vi "CreateErrorControls.vi"(8 "error in (no error)":errorcluster, 11 "VI in":refnum<vi>) -> (0 "error out":errorcluster, 2 "Control terminals on top-level":refnum<vi>[](array[refnum]), 3 "VI out (dup)":refnum<vi>, 4 "Error terminals":T1)   [LabVIEW 2017, in "ErrorStructureDrawer.lvlib"]
doc: "Checks if an error control and error indicator exist. If so, gets a reference to it/them. Otherwise, creates and positions (within front panel) an error control and/or error indicator."
uses:
  ErrorStructureDrawer.lvlib
  Controls/ErrorTerminals.ctl
  <vilib>/Utility/traverseref.llb/TRef TravTarget.ctl
  <vilib>/Utility/miscctls.llb/LVPointTypeDef.ctl
  <vilib>/Utility/miscctls.llb/LVPositionTypeDef.ctl
  GetErrorControlVertSpacingFP.vi
  GetErrorControlPath.vi
  GetErrorControlHorizSpacingFP.vi
  GetErrorIndicatorPath.vi
  <vilib>/Utility/traverseref.llb/VI Scripting - Traverse.lvlib
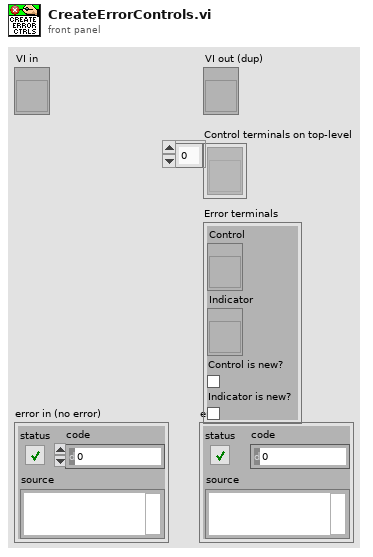
[diagram p1: front panel]
types:
  T1 = typedef "ErrorStructureDrawer.lvlib/ErrorTerminals.ctl" = cluster{"Control":refnum<vi>, "Indicator":refnum<vi>, "Control is new?":bool, "Indicator is new?":bool}
  T2 = typedef "LVPositionTypeDef.ctl" = cluster{"Left":i32, "Top":i32}
  T3 = typedef "LVPointTypeDef.ctl" = cluster{"Horizontal":i16, "Vertical":i16}
  T4 = typedef "TRef TravTarget.ctl" = enum16{"FP", "BD", "Other"}
  T5 = typedef "LVBoundsTypeDef.ctl" = cluster{"Width":u32, "Height":u32}
  T6 = typedef "LVRectTypeDef.ctl" = cluster{"Left":i16, "Top":i16, "Right":i16, "Bottom":i16}
  T7 = cluster{"Left":i32, "Top":i32, "Right":i32, "Bottom":i32}
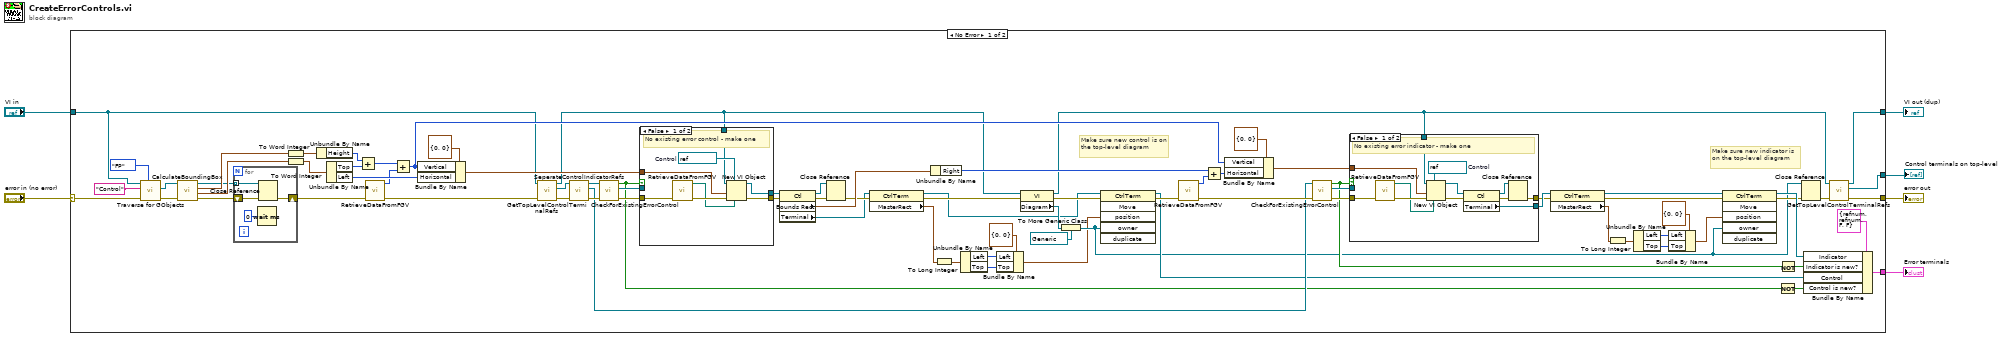
[diagram p0: block diagram]
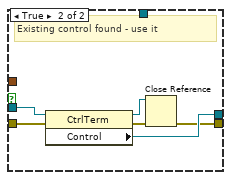
[diagram p3: hidden frame]
diagram:
  n1 = case shown="No Error" "error in (no error)" {
    selector: "error in (no error)" -> [w56 w122]
    tunnel: "VI in" -> [w50 w121]
    tunnel: [w59 w122] -> w5
    tunnel: [w63 _] -> w4
    tunnel: [w57 w121] -> w2
    tunnel: [w58 _] -> w1
    frame No Error {
      # "Make sure new indicator is on the top-level diagram"
      # "Make sure new control is on the top-level diagram"
      n2 = call <vilib>:"Traverse for GObjects.vi"("Traverse Target"=TRef_TravTarget."FP", "error in (no error)"=w56, "Class Name"="Control", "VI Refnum"=w50) -> ("error out"=w71:errorcluster, "References"=w86:refnum<vi>[])  [unwired: 4 in, 2 out]
      n3 = call "CalculateBoundingBox.vi"("error in (no error)"=w71, "Items"=w86) -> ("error out"=w67:errorcluster, "Current bounding box position"=w80:cluster{"Left":i32, "Top":i32}, "Size of bounding box for items"=w82:T5, "Items out (dup)"=w68:refnum<vi>[])  [unwired: 6 in]
      n4 = for {
        tunnel: w68 -> [w120] mode=indexing
        shift-right: [w118] -> w60
        shift-left: w67 -> [w119]
        n5 = Wait (ms)(milliseconds to wait=u32 0) -> ()  [unwired: 1 out]
        n6 = Close Reference(reference=w120, error in (no error)=w119) -> (error out=w118:errorcluster)
      }
      n7 = To Word Integer(number=w82) -> (16bit integer=w81:cluster{"Width":i16, "Height":i16})
      n8 = To Word Integer(number=w80) -> (16bit integer=w79:cluster{"Left":i16, "Top":i16})
      n9 = Unbundle By Name(w81) -> ("Height"=w83:i16)
      n10 = Unbundle By Name(w79) -> ("Top"=w78:i16, "Left"=w77:i16)
      n11 = Add(x=w83, y=w78) -> (x+y=w76:i16)
      n12 = call-poly "RetrieveDataFromFGV.vi"("error in (no error)"=w60) -> ("error out"=w51:errorcluster, "Error control vertical spacing from existing FP items"=w61:i16)  [unwired: 9 in]
      n13 = Add(x=w76, y=w61) -> (x+y=w72:i16)
      n14 = Bundle By Name(cluster=T3 {"Horizontal"=0, "Vertical"=0} ("location"), "Vertical"=w72, "Horizontal"=w77) -> (w84:T3)
      n15 = call "GetTopLevelControlTerminalRefs.vi"("error in (no error)"=w51, "VI ref in"=w50) -> ("error out"=w55:errorcluster, "Control terminals on top-level"=w54:refnum<vi>[], "VI ref out (dup)"=w35:refnum<vi>)  [unwired: 7 in]
      n16 = call "SeperateControlIndicatorRefs.vi"("error in (no error)"=w55, "Terminal references"=w54) -> ("error out"=w53:errorcluster, "Indicator references"=w43:refnum<vi>[], "Control references"=w52:refnum<vi>[])  [unwired: 7 in]
      n17 = call "CheckForExistingErrorControl.vi"("error in (no error)"=w53, "Control terminals to check"=w52) -> ("error out"=w49:errorcluster, "Error control ref"=w48:refnum<vi>, "Error control found?"=w42:bool)  [unwired: 7 in]
      n18 = case shown="False" w42 {
        tunnel: w84 -> [w109 _]
        tunnel: [w108 w114] -> w75
        tunnel: [w107 w112] -> w70
        tunnel: w49 -> [w104 w116]
        tunnel: w35 -> [w103 _]
        tunnel: w48 -> [_ w115]
        frame False {
          w110 = refnum<vi> refnum  # Control
          # "No existing error control - make one"
          n19 = call-poly "RetrieveDataFromFGV.vi"("error in (no error)"=w104) -> ("error out"=w106:errorcluster, "Error control path"=w105:path)  [unwired: 9 in]
          n20 = New VI Object(vi object class=w110, owner refnum=w103, position/next to=w109, 6:w105, 8:w106) -> (object refnum=w108:refnum<vi>, 0:w107:errorcluster)  [unwired: 3 in]
        }
        frame True {
          # "Existing control found - use it"
          n21 = property class="CtrlTerm"(reference=w115, error in=w116) -> (reference out=w111:refnum<vi>, error out=w113:errorcluster, "Control"=w114:refnum<vi>)
          n22 = Close Reference(reference=w111, error in (no error)=w113) -> (error out=w112:errorcluster)
        }
      }
      n23 = property class="Ctl"(reference=w75, error in=w70) -> (reference out=w65:refnum<vi>, error out=w66:errorcluster, "Bounds Rect"=w22:T6, "Terminal"=w10:refnum<vi>)
      n24 = Close Reference(reference=w65, error in (no error)=w66) -> (error out=w11:errorcluster)
      n25 = property class="CtrlTerm"(reference=w10, error in=w11) -> (reference out=w7:refnum<vi>, error out=w8:errorcluster, "MasterRect"=w9:T6)
      n26 = Unbundle By Name(w22) -> ("Right"=w47:i16)
      n27 = To Long Integer(number=w9) -> (32bit integer=w23:T7)
      n28 = Unbundle By Name(w23) -> ("Left"=w25:i32, "Top"=w24:i32)
      n29 = Bundle By Name(cluster=T2 {"Left"=0, "Top"=0} ("position"), "Left"=w25, "Top"=w24) -> (w26:T2)
      n30 = property class="VI"(reference=w35, error in=w8) -> (reference out=w34:refnum<vi>, error out=w36:errorcluster, "Diagram"=w33:refnum<vi>)
      n31 = To More Generic Class(target class=refnum<vi> refnum ("owner"), reference=w33) -> (generic class reference=w28:refnum<vi>)
      n32 = invoke class="CtrlTerm" method="Move"(reference=w7, error in=w36, "position"=w26, "owner"=w28) -> (reference out=w37:refnum<vi>, error out=w38:errorcluster)  [unwired: 2 in, 4 out]
      n33 = call-poly "RetrieveDataFromFGV.vi"("error in (no error)"=w38) -> ("error out"=w46:errorcluster, "Error control-indicator horizontal spacing on FP"=w62:i16)  [unwired: 9 in]
      n34 = Add(x=w47, y=w62) -> (x+y=w69:i16)
      n35 = Bundle By Name(cluster=T3 {"Horizontal"=0, "Vertical"=0} ("location"), "Vertical"=w72, "Horizontal"=w69) -> (w73:T3)
      n36 = call "CheckForExistingErrorControl.vi"("error in (no error)"=w46, "Control terminals to check"=w43) -> ("error out"=w45:errorcluster, "Error control ref"=w44:refnum<vi>, "Error control found?"=w40:bool)  [unwired: 7 in]
      n37 = case shown="False" w40 {
        tunnel: w73 -> [w98 _]
        tunnel: [w94 w101] -> w21
        tunnel: w45 -> [w91 w102]
        tunnel: [w90 w102] -> w20
        tunnel: w34 -> [w89 _]
        tunnel: w44 -> [_ w101]
        frame False {
          w100 = refnum<vi> refnum  # Control
          # "No existing error indicator - make one"
          n38 = call-poly "RetrieveDataFromFGV.vi"("error in (no error)"=w91) -> ("error out"=w93:errorcluster, "Error indicator path"=w92:path)  [unwired: 9 in]
          n39 = New VI Object(vi object class=w100, owner refnum=w89, position/next to=w98, 6:w92, 8:w93) -> (object refnum=w96:refnum<vi>, 0:w99:errorcluster)  [unwired: 3 in]
          n40 = property class="Ctl"(reference=w96, error in=w99) -> (reference out=w95:refnum<vi>, error out=w97:errorcluster, "Terminal"=w94:refnum<vi>)
          n41 = Close Reference(reference=w95, error in (no error)=w97) -> (error out=w90:errorcluster)
        }
        frame True {
          # "Existing indicator found - use it"
        }
      }
      n42 = property class="CtrlTerm"(reference=w21, error in=w20) -> (reference out=w19:refnum<vi>, error out=w18:errorcluster, "MasterRect"=w12:T6)
      n43 = To Long Integer(number=w12) -> (32bit integer=w15:T7)
      n44 = Unbundle By Name(w15) -> ("Left"=w17:i32, "Top"=w16:i32)
      n45 = Bundle By Name(cluster=T2 {"Left"=0, "Top"=0} ("position"), "Left"=w17, "Top"=w16) -> (w13:T2)
      n46 = invoke class="CtrlTerm" method="Move"(reference=w19, error in=w18, "position"=w13, "owner"=w28) -> (reference out=w31:refnum<vi>, error out=w30:errorcluster)  [unwired: 2 in, 4 out]
      n47 = Not(x=w42) -> (.not. x?=w41:bool)
      n48 = Not(x=w40) -> (.not. x?=w39:bool)
      n49 = Close Reference(reference=w28, error in (no error)=w30) -> (error out=w29:errorcluster)
      n50 = Bundle By Name(cluster=T1 {"Control"=refnum, "Indicator"=refnum, "Control is new?"=FALSE, "Indicator is new?"=FALSE} ("Error terminals"), "Indicator"=w31, "Indicator is new?"=w39, "Control"=w37, "Control is new?"=w41) -> (w63:T1)
      n51 = call "GetTopLevelControlTerminalRefs.vi"("error in (no error)"=w29, "VI ref in"=w34) -> ("error out"=w59:errorcluster, "Control terminals on top-level"=w58:refnum<vi>[], "VI ref out (dup)"=w57:refnum<vi>)  [unwired: 7 in]
    }
    frame Error {
    }
  }
  "error out" <- w5
  "VI out (dup)" <- w2
  "Error terminals" <- w4
  "Control terminals on top-level" <- w1
